vi "open.vi"(8 "error in (no error)":errorcluster, 11 "Instrument in":refnum<class "PZT.lvclass">) -> (0 "error out":errorcluster, 3 "Instrument out":refnum<class "PZT.lvclass">)   [LabVIEW 2020, in "PZT.lvclass"]
uses:
  PZT.lvclass
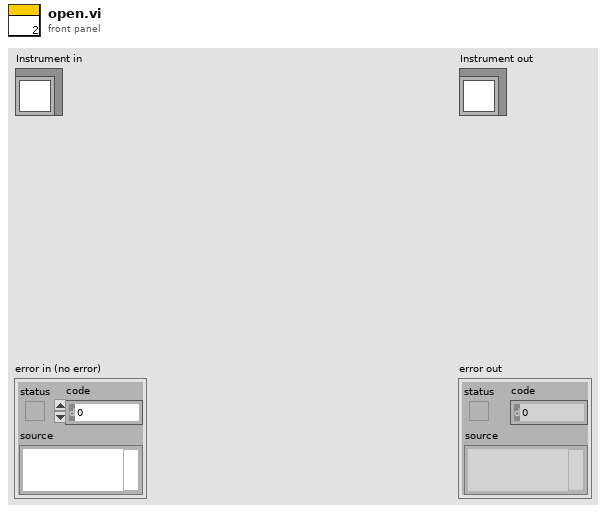
[diagram p1: front panel]
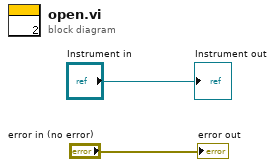
[diagram p0: block diagram]
diagram:
  "error out" <- "error in (no error)"
  "Instrument out" <- "Instrument in"
